vi "PXI_Host_Cluster_Write_NewMethod_Benchmark.vi"() -> ()   [LabVIEW 2018]
uses:
  cRIO RT/TypeDefs/Simple cluster.ctl
  4e6a3d45-ffd6-4a6c-bc5a-fe382907064f.vi
  4e6a3d45-ffd6-4a6c-bc5a-fe382907064f.vi/b5ba7d49-12fb-406f-82d8-b5daff98c8fb.vi
  cRIO RT/FPGA Bitfile Register Operations/Scalar IO Operations/SubVIs/Parse Cluster Configuration.vi
  cRIO RT/FPGA Bitfile Register Operations/Scalar IO Operations/SubVIs/DBL to FXP Raw.vi
  cRIO RT/FPGA Bitfile Register Operations/Scalar IO Operations/SubVIs/Convert Bool Array to Cluster BLOB.vi
  cRIO RT/FPGA Bitfile Register Operations/Scalar IO Operations/Write Methods/Write Data Register/Instances/Write U8 Array.vi
  <vilib>/FPGAPlugInAG/Dynamic/niLvFpga_Close_Dynamic.vi
  <vilib>/rvi/interface/nirviCloseFPGA/nirviCloseFPGA.xnode
  cRIO RT/FPGA Bitfile Register Operations/Scalar IO Operations/FPGA Register IO.lvlib
panel:
  out "error out":errorcluster
  out "Value out":T1
  out "Execution time (s)":dbl
  # "Recorded time"
  # "3.37551E-5"
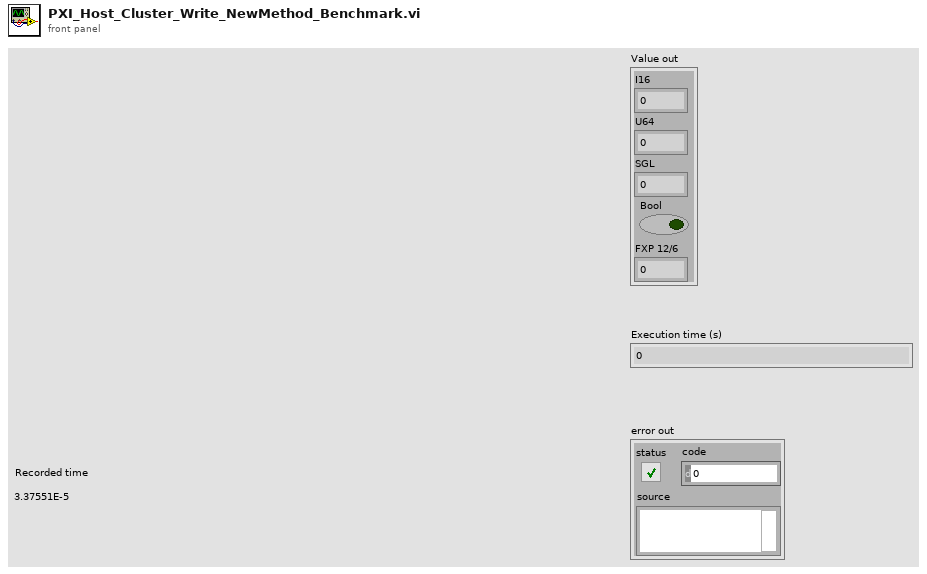
[diagram p1: front panel]
types:
  T1 = typedef "Simple cluster.ctl" = cluster{"I16":i16, "U64":u64, "SGL":sgl, "Bool":bool, "FXP 12/6":fxp<+/-,12,6>}
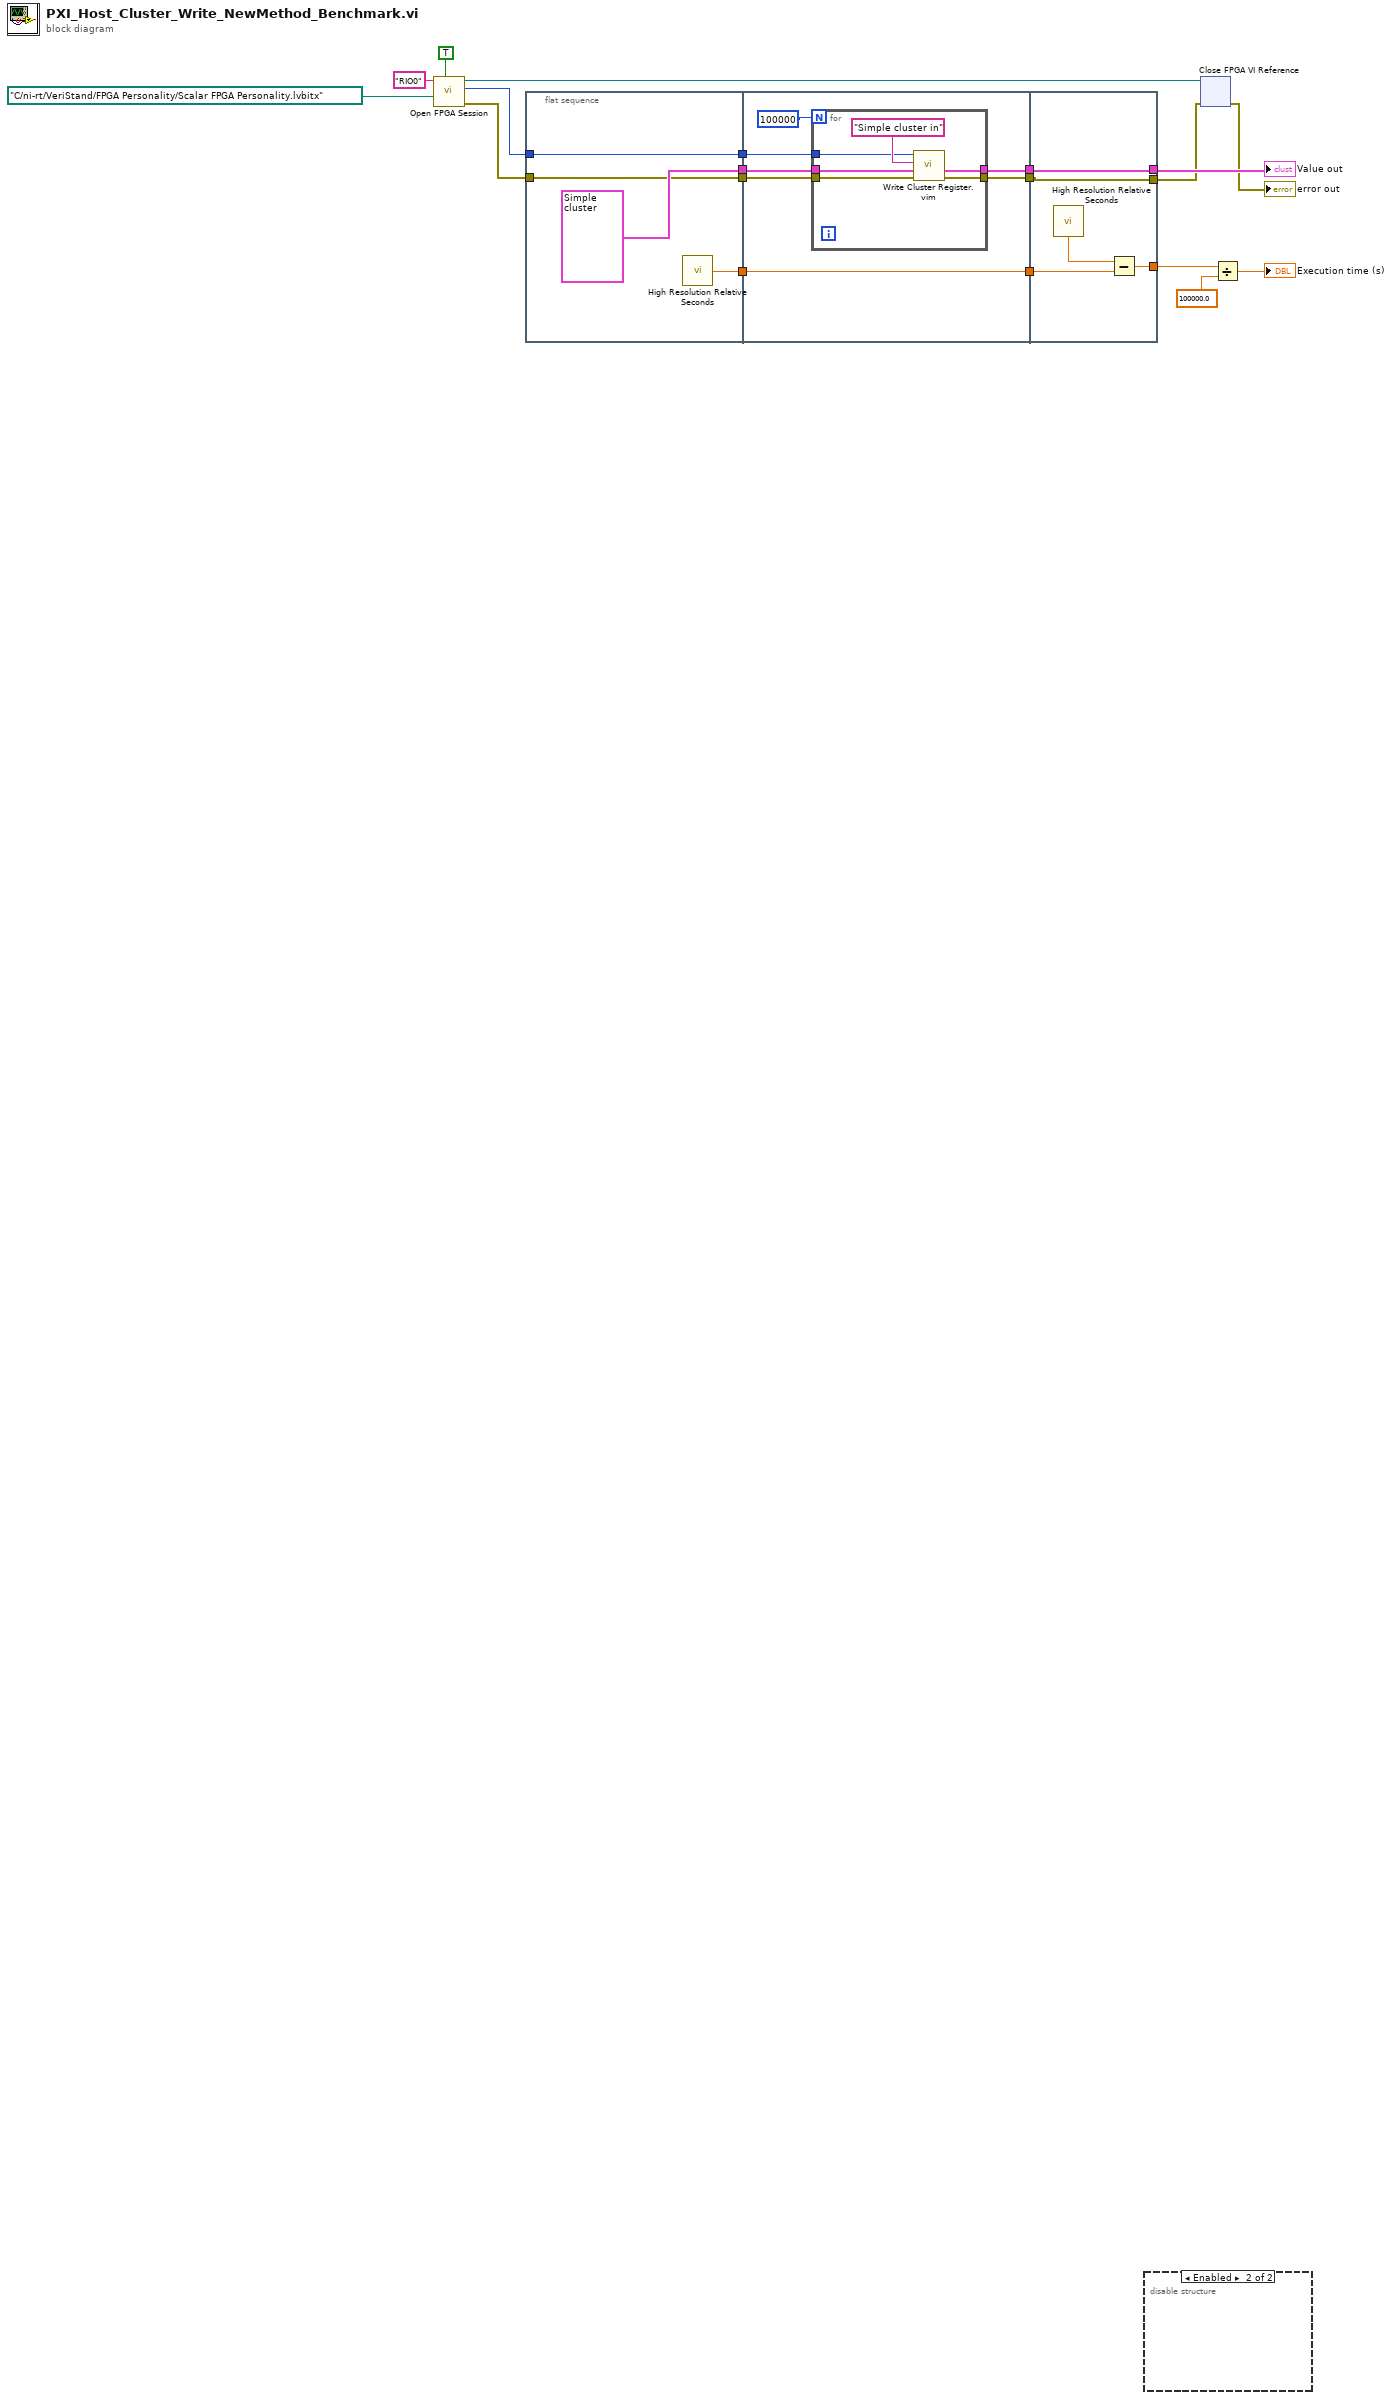
[diagram p0: block diagram]
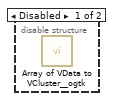
[diagram p2: hidden frame]
diagram:
  n1 = call "Open FPGA Session.vi"("run when loaded (T)"=TRUE, "bitfile path"=path "C:/ni-rt/VeriStand/FPGA Personality/Scalar FPGA Personality.lvbitx", "device address"="RIO0") -> ("error out"=w7:errorcluster, "session out"=w12:u32, "bitfile reference out"=w3:refnum<k20>)  [unwired: 6 in]
  n2 = flat-sequence {
    tunnel: [T1 {"I16"=1231, "U64"=213123, "SGL"=1.0, "Bool"=TRUE, "FXP 12/6"=31.984375} ("Simple Cluster")] -> w19
    tunnel: [w22] -> w17
    tunnel: w12 -> [w21]
    tunnel: [w21] -> w11
    tunnel: w7 -> [w20]
    tunnel: [w20] -> w6
    tunnel: w19 -> [w29]
    tunnel: [w28] -> w18
    tunnel: w17 -> [w28]
    tunnel: [w27] -> w13
    tunnel: w11 -> [w26]
    tunnel: w6 -> [w25]
    tunnel: [w24] -> w5
    tunnel: w18 -> [w40]
    tunnel: [w39] -> w16
    tunnel: w13 -> [w37]
    tunnel: w5 -> [w38]
    tunnel: [w38] -> w2
    tunnel: [w37] -> w4
    frame #0 {
      n3 = call <vilib>:"High Resolution Relative Seconds.vi"() -> ("relative seconds"=w22:dbl)
    }
    frame #1 {
      n4 = for {
        N: 100000 -> [_]
        tunnel: w29 -> [w36]
        tunnel: [w34] -> w27
        tunnel: w26 -> [w33]
        tunnel: w25 -> [w32]
        tunnel: [w31] -> w24
        n5 = call "Write Cluster Register.vim"("error in (no error)"=w32, "Cluster in (default value)"=w36, "Cluster Name"="Simple cluster in", "session in"=w33) -> ("error out"=w31:errorcluster, "Cluster out"=w34:T1)  [unwired: 5 in, 1 out]
      }
    }
    frame #2 {
      n6 = call <vilib>:"High Resolution Relative Seconds.vi"() -> ("relative seconds"=w41:dbl)
      n7 = Subtract(x=w41, y=w40) -> (x-y=w39:dbl)
    }
  }
  n8 = disable-structure shown="Enabled" {
    frame Disabled {
      n9 = call <userlib>:"Array of VData to VCluster__ogtk.vi"() -> ()  [unwired: 10 in, 2 out]
    }
    frame Enabled {
    }
  }
  n10 = xnode "Close FPGA VI Reference"("FPGA VI Reference In"=w3, "error in"=w2) -> ("error out"=→"error out":errorcluster)
  n11 = Divide(x=w16, y=100000.0) -> (x/y=→"Execution time (s)":dbl)
  "Value out" <- w4
